vi "Set Output Value.vi"(8 "Error In":errorcluster, 9 "Channel":i32, 10 "Value":dbl, 11 "BNT_DAQmx-MCSV in":refnum<class "BNT_DAQmx-MCSV.lvclass">) -> (0 "Error Out":errorcluster, 3 "BNT_DAQmx-MCSV out":refnum<class "BNT_DAQmx-MCSV.lvclass">)   [LabVIEW 2019, in "BNT_DAQmx.lvlib" / "BNT_DAQmx-MCSV.lvclass"]
doc: "Write voltage values to DAQmx device and publish.\n\nTimeout is set to constant 1s."
uses:
  BNT_DAQmx-MCSV.lvclass
  BNT_DAQmx-MCSV.lvclass/BNT_DAQmx-MCSV.ctl
  <vilib>/DAQmx/write.llb/DAQmx Write (Analog 1D DBL NChan 1Samp).vi
  <vilib>/DAQmx/miscellaneous.llb/DAQmx Fill In Error Info.vi
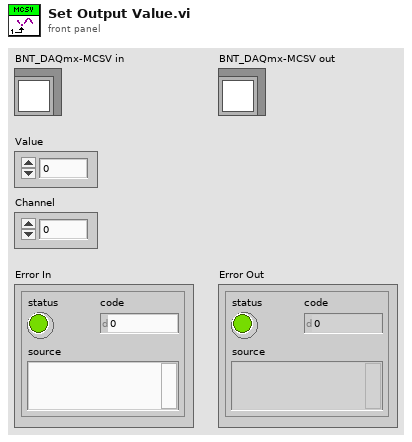
[diagram p1: front panel]
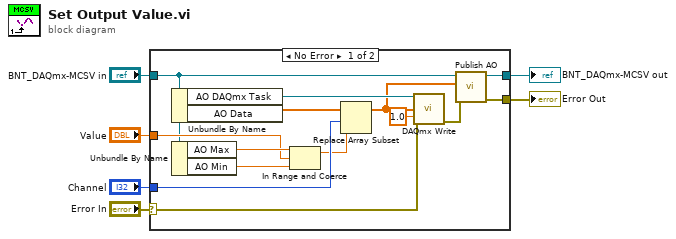
[diagram p0: block diagram]
diagram:
  n1 = case shown="No Error" "Error In" {
    selector: "Error In" -> [w18 w22]
    tunnel: [w9 w22] -> w5
    tunnel: [w10 w21] -> w3
    tunnel: "BNT_DAQmx-MCSV in" -> [w11 w21]
    tunnel: "Value" -> [w15 _]
    tunnel: "Channel" -> [w13 _]
    frame No Error {
      n2 = Unbundle By Name(w11) -> ("AO DAQmx Task"=w20:refnum<k21>, "AO Data"=w14:dbl[])
      n3 = Unbundle By Name(w11) -> ("AO Max"=w17:dbl, "AO Min"=w16:dbl)
      n4 = In Range and Coerce(upper limit=w17, x=w15, lower limit=w16) -> (coerced(x)=w12:dbl)  [unwired: 1 out]
      n5 = Replace Array Subset(array=w14, new element=w12, index=w13) -> (w8:dbl[])
      n6 = call-poly <vilib>:"DAQmx Write.vi"("task/channels in"=w20, "data"=w8, "timeout"=1.0, "error in"=w18) -> ("error out"=w7:errorcluster)  [unwired: 9 in, 2 out]
      n7 = call "Publish AO.vi"("error in"=w7, "AO Data"=w8, "BNT_DAQmx-MCSV in"=w11) -> ("error out"=w9:errorcluster, "BNT_DAQmx-MCSV out"=w10:refnum<class "BNT_DAQmx-MCSV.lvclass">)  [unwired: 7 in]
    }
    frame Error {
    }
  }
  "Error Out" <- w5
  "BNT_DAQmx-MCSV out" <- w3
